vi "Create One Timeset.vi"(6 "Timeset Name":string="-", 7 "Notes":string, 8 "error in (no error)":errorcluster, 9 "PinStates":T1[](array[typedef]), 10 "OpCode":string, 11 "SPI 4W Pattern Creator in":refnum<class "SPI 4W Pattern Creator.lvclass">) -> (0 "error out":errorcluster, 2 "String  out":string, 3 "SPI 4W Pattern Creator out":refnum<class "SPI 4W Pattern Creator.lvclass">)   [LabVIEW 2018, in "SPI 4W Pattern Creator.lvlib" / "SPI 4W Pattern Creator.lvclass"]
uses:
  SPI 4W Pattern Creator.lvclass
  Interfaces/Protocol Interface.lvlibp/Interfaces/Protocol Interface/Pin State.ctl
  Interfaces/Protocol Interface.lvlibp/Interfaces/Protocol Interface/Protocol Interface.lvclass
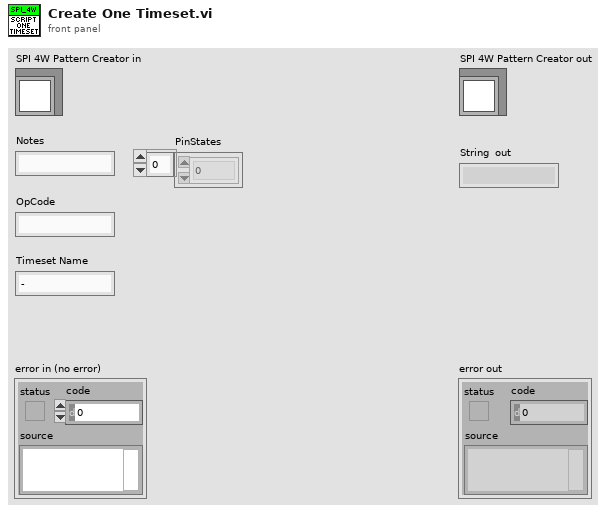
[diagram p1: front panel]
types:
  T1 = typedef "Protocol Interface.lvlibp/Protocol Interface.lvclass/Pin State.ctl" = enum16{"0", "1", "L", "H", "X", "V", "D", "M"}
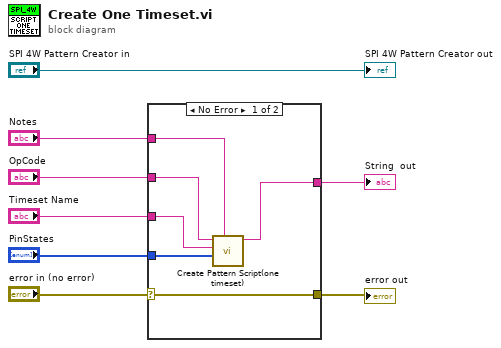
[diagram p0: block diagram]
diagram:
  n1 = case shown="No Error" "error in (no error)" {
    selector: "error in (no error)" -> [w9 w15]
    tunnel: "Notes" -> [w14 _]
    tunnel: "OpCode" -> [w13 _]
    tunnel: "Timeset Name" -> [w12 _]
    tunnel: "PinStates" -> [w11 _]
    tunnel: [w10 _] -> w4
    tunnel: [w9 w15] -> w1
    frame No Error {
      n2 = call "Create Pattern Script(one timeset).vi"("Notes"=w14, "Pin States"=w11, "timeset name"=w12, "opcode"=w13) -> ("string out"=w10:string)  [unwired: 7 in]
    }
    frame Error {
    }
  }
  "error out" <- w1
  "String  out" <- w4
  "SPI 4W Pattern Creator out" <- "SPI 4W Pattern Creator in"
